vi "CRC16.vi"(1 "CRC IN":string) -> (0 "CRC Out":string)   [LabVIEW 2021]
panel:
  out "length of CRC":i32
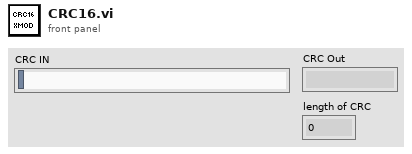
[diagram p1: front panel]
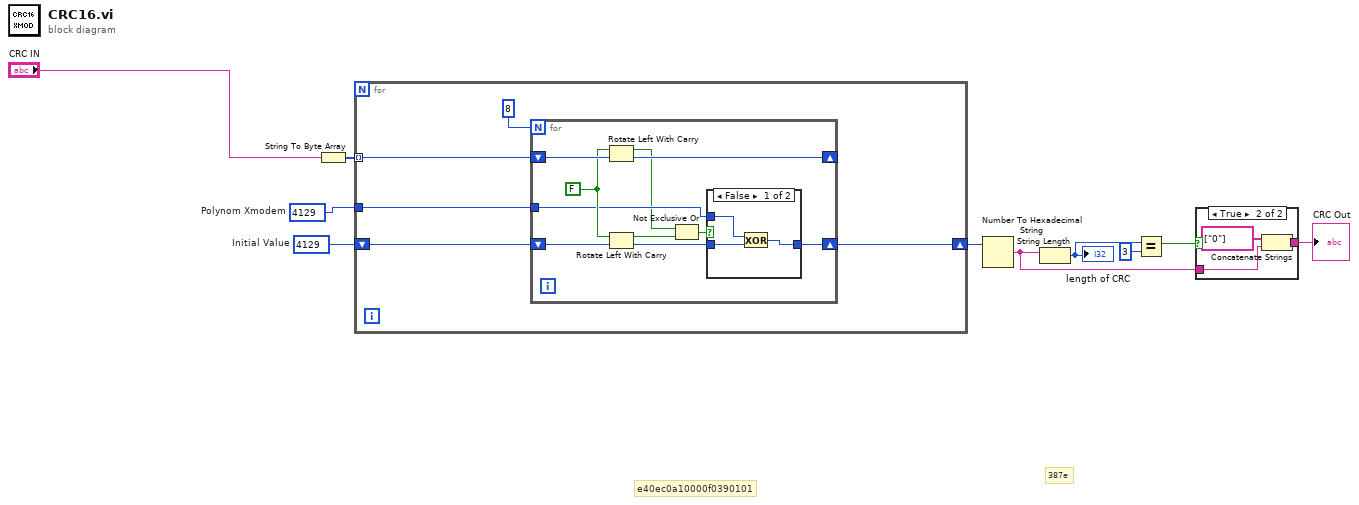
[diagram p0: block diagram]
diagram:
  w9 = u16 4129  # Polynom Xmodem
  w10 = u16 4129  # Initial Value
  # "387e"
  # "e40ec0a10000f0390101"
  n1 = String To Byte Array(string="CRC IN") -> (unsigned byte array=w8:u8[])
  n2 = for {
    tunnel: w8 -> [w14] mode=indexing
    shift-right: [w12] -> w3
    shift-left: w10 -> [w13]
    tunnel: w9 -> [w11]
    n3 = for {
      N: 8 -> [_]
      shift-right: [w22] -> w12
      shift-left: w13 -> [w25]
      shift-right: [w23] -> _
      shift-left: w14 -> [w24]
      tunnel: w11 -> [w19]
      w20 = FALSE
      n4 = Rotate Left With Carry(2:w24, 3:w20) -> (0:w23:u8, 1:w16:bool)
      n5 = Rotate Left With Carry(2:w25, 3:w20) -> (0:w21:u16, 1:w17:bool)
      n6 = Not Exclusive Or(1:w17, 2:w16) -> (0:w18:bool)
      n7 = case shown="False" w18 {
        tunnel: [w26 w29] -> w22
        tunnel: w21 -> [w28 w29]
        tunnel: w19 -> [w27 _]
        frame False {
          n8 = Exclusive Or(1:w28, 2:w27) -> (0:w26:u16)
        }
        frame True {
        }
      }
    }
  }
  n9 = Number To Hexadecimal String(2:w3) -> (0:w2:string)  [unwired: 1 in]
  n10 = String Length(string=w2) -> (length=w7:i32)
  "length of CRC" <- w7
  n11 = Equal?(x=w7, y=3) -> (x = y?=w5:bool)
  n12 = case shown="True" w5 {
    tunnel: [w30 w33] -> w4
    tunnel: w2 -> [w30 w31]
    frame False {
    }
    frame True {
      n13 = Concatenate Strings(string[] ["0"] ("string"), w31) -> (w33:string)
    }
  }
  "CRC Out" <- w4
